vi "Test 3 Get Heat in Col from Down.vi"(8 "error in (no error)":errorcluster, 11 "Test Case In":refnum<class "Tests.lvclass">) -> (0 "error out":errorcluster, 3 "Test Case Out":refnum<class "Tests.lvclass">)   [LabVIEW 2021, in "Tests.lvclass"]
uses:
  Tests.lvclass
  Tests.lvclass/Tests.ctl
  4993e8ee-a06a-463a-9684-69129f64d5ce.vi
  Proto/Proto.lvclass
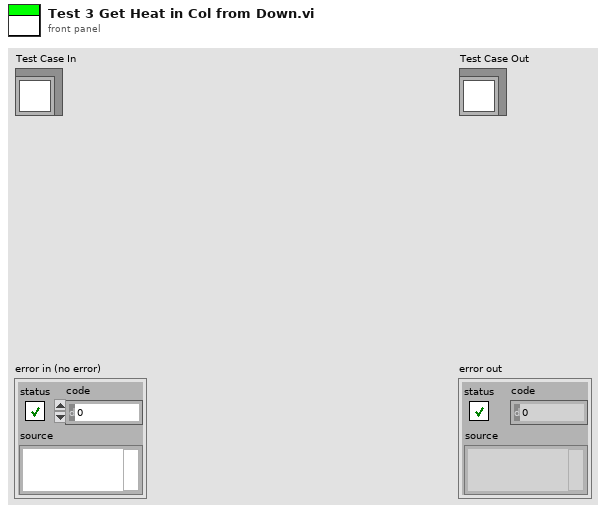
[diagram p1: front panel]
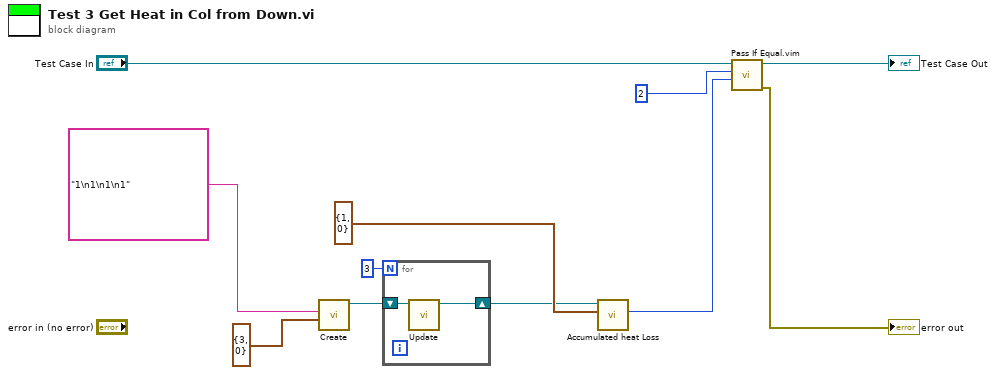
[diagram p0: block diagram]
diagram:
  n1 = call "Create.vi"("Start Position"=cluster{"Row":i32, "Col":i32} {"Row"=3, "Col"=0}, "Input"="1\n1\n1\n1") -> ("Proto"=w8:refnum<class "Proto.lvclass">)  [unwired: 9 in]
  n2 = for {
    N: 3 -> [_]
    shift-right: [w12] -> w2
    shift-left: w8 -> [w13]
    n3 = call "Update.vi"("Proto in"=w13) -> ("Proto out"=w12:refnum<class "Proto.lvclass">)  [unwired: 9 in, 1 out]
  }
  n4 = call "Accumulated heat Loss.vi"("Coord"=cluster{"Row":i32, "Col":i32} {"Row"=1, "Col"=0}, "Proto in"=w2) -> ("Min Heat"=w5:i32)  [unwired: 8 in, 1 out]
  n5 = call "Pass If Equal.vim"("Actual"=w5, "Expected"=2 ("Heat"), "LUnit Test Case In"="Test Case In") -> ("error out"=→"error out":errorcluster, "LUnit Test Case Out"=→"Test Case Out":refnum<class "Tests.lvclass">)  [unwired: 7 in]
